vi "Configure Active Compliance.vi"(8 "error in (no error)":errorcluster, 9 "Active Compliance Settings":T1={"Clockwise Slope (9.38416 deg)"=9.384164, "Counter-Clockwise Slope (9.38416 deg)"=9.384164, "Clockwise Margin (0.293255 deg)"=0.29325512, "Counter-Clockwise Margin (0.293255 deg)"=0.29325512, "Punch (0%)"=0.0, "Max  Torque (100%)"=100.0}, 10 "Motor ID (0)":u8, 11 "VISA resource name":refnum<visa-resource-name>) -> (0 "error out":errorcluster, 3 "VISA resource name out":refnum<visa-resource-name>)   [LabVIEW 2016, in "Dynamixel Motor.lvlib"]
doc: "Adjusts the active compliance of the motor. See the motor's user manual for more details."
uses:
  Dynamixel Motor.lvlib
  Active Compliance Settings.ctl
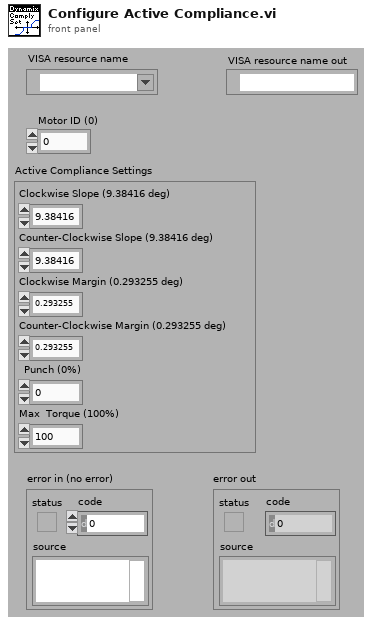
[diagram p1: front panel]
types:
  T1 = typedef "Dynamixel Motor.lvlib/Active Compliance Settings.ctl" = cluster{"Clockwise Slope (9.38416 deg)":sgl, "Counter-Clockwise Slope (9.38416 deg)":sgl, "Clockwise Margin (0.293255 deg)":sgl, "Counter-Clockwise Margin (0.293255 deg)":sgl, "Punch (0%)":sgl, "Max  Torque (100%)":sgl}
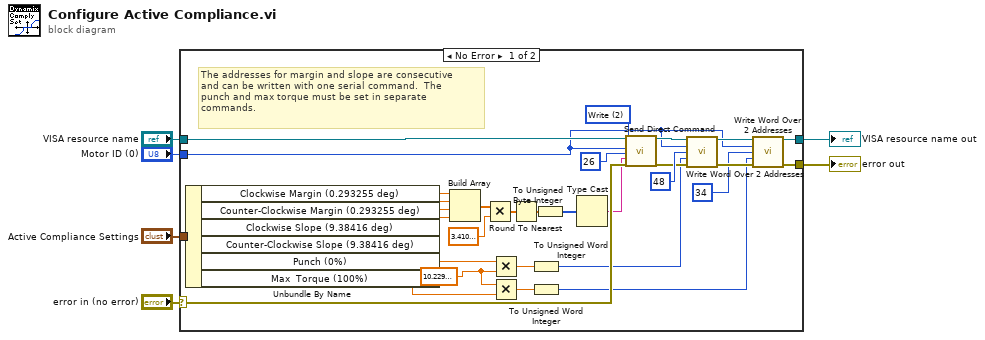
[diagram p0: block diagram]
diagram:
  n1 = case shown="No Error" "error in (no error)" {
    selector: "error in (no error)" -> [w29 w39]
    tunnel: "VISA resource name" -> [w37 w38]
    tunnel: "Motor ID (0)" -> [w24 _]
    tunnel: "Active Compliance Settings" -> [w36 _]
    tunnel: [w20 w39] -> w2
    tunnel: [w21 w38] -> w1
    frame No Error {
      w11 = sgl 10.23 ("y")
      w31 = u16 2 items=["Ping", "Read", "Write", "Registered Write", "Action", "Reset", "Sync Write"] ("Select Action")
      # "The addresses for margin and slope are consecutive \nand can be written with one serial command.  The\npunch and max torque must be set in separate\ncommands."
      n2 = Unbundle By Name(w36) -> ("Clockwise Margin (0.293255 deg)"=w35:sgl, "Counter-Clockwise Margin (0.293255 deg)"=w34:sgl, "Clockwise Slope (9.38416 deg)"=w33:sgl, "Counter-Clockwise Slope (9.38416 deg)"=w32:sgl, "Punch (0%)"=w13:sgl, "Max  Torque (100%)"=w12:sgl)
      n3 = Build Array(w35, w34, w33, w32) -> (w18:sgl[])
      n4 = Multiply(x=w18, y=sgl 3.41) -> (x*y=w16:sgl[])
      n5 = Multiply(x=w13, y=w11) -> (x*y=w10:sgl)
      n6 = Multiply(x=w11, y=w12) -> (x*y=w9:sgl)
      n7 = Round To Nearest(number=w16) -> (nearest integer value=w15:sgl[])
      n8 = To Unsigned Word Integer(number=w10) -> (unsigned 16bit integer=w8:u16)
      n9 = To Unsigned Word Integer(number=w9) -> (unsigned 16bit integer=w7:u16)
      n10 = To Unsigned Byte Integer(number=w15) -> (unsigned 8bit integer=w14:u8[])
      n11 = Type Cast(x=w14) -> (*(type *) &x=w19:string)  [unwired: 1 in]
      n12 = call "Send Direct Command.vi"("VISA resource name"=w37, "Select Action"=w31, "Motor ID (0)"=w24, "Address"=u8 26, "Parameters"=w19, "Error in (no error)"=w29) -> ("VISA resource name out"=w28:refnum<visa-resource-name>, "Error out"=w26:errorcluster)  [unwired: 11 in, 1 out]
      n13 = call "Write Word Over 2 Addresses.vi"("VISA resource name"=w28, "Motor ID (0)"=w24, "Address number (0)"=u8 48, "Parameter (0)"=w8, "error in (no error)"=w26) -> ("VISA resource name out"=w25:refnum<visa-resource-name>, "error out"=w23:errorcluster)  [unwired: 9 in]
      n14 = call "Write Word Over 2 Addresses.vi"("VISA resource name"=w25, "Motor ID (0)"=w24, "Address number (0)"=u8 34 ("Address"), "Parameter (0)"=w7, "error in (no error)"=w23) -> ("VISA resource name out"=w21:refnum<visa-resource-name>, "error out"=w20:errorcluster)  [unwired: 9 in]
    }
    frame Error {
    }
  }
  "VISA resource name out" <- w1
  "error out" <- w2
